vi "LJUD U3RAW Reset.vi"(7 "Comm Settings":T1={"Open LabJack "=TRUE, "Address"="1", "FirstFound"=TRUE}, 8 "error in (no error)":errorcluster, 11 "Handle In":i32) -> (0 "error out":errorcluster, 3 "Handle Out":i32)   [LabVIEW 2021]
panel:
  in  "Hard Reset":bool=TRUE
  in  "Soft Reset":bool
  out "Read Array":u8[](array[numeric]) format="%.0x"
  # "If open is false,\nthen a valid\nhandle must be\npassed in."
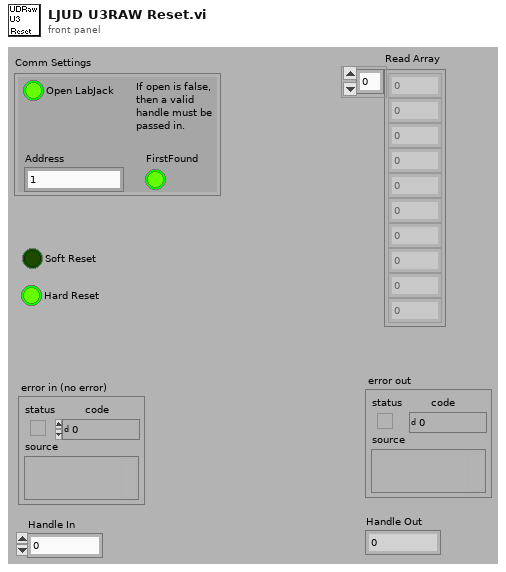
[diagram p1: front panel]
types:
  T1 = cluster{"Open LabJack ":bool, "Address":string, "FirstFound":bool}
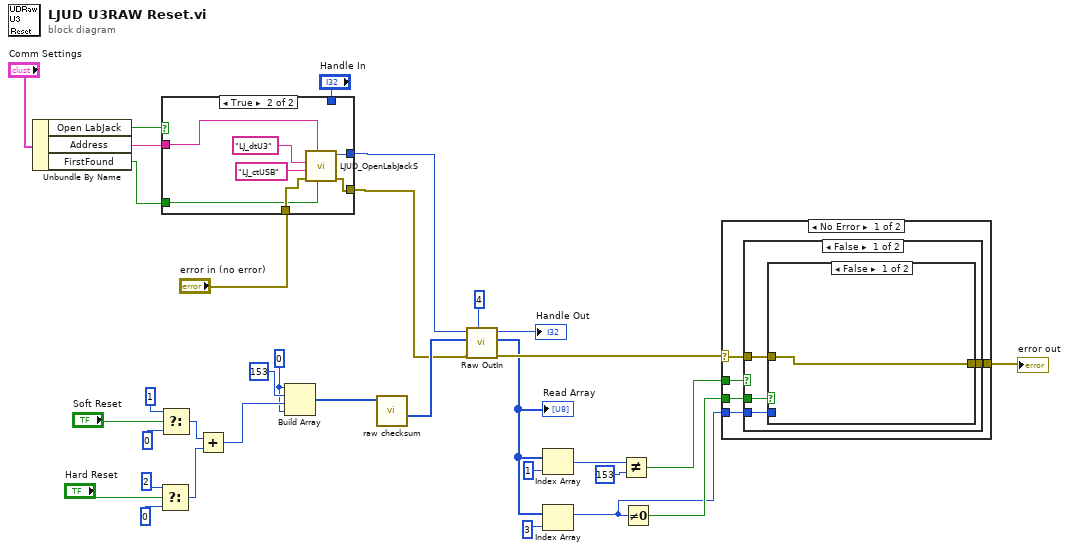
[diagram p0: block diagram]
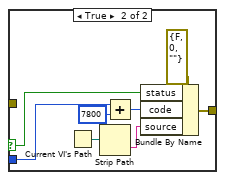
[diagram p2: hidden frame]
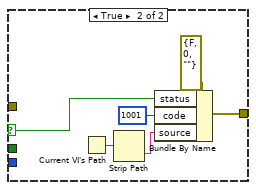
[diagram p3: hidden frame]
diagram:
  w9 = u8 0 ("Input Element")
  n1 = Unbundle By Name("Comm Settings") -> ("Open LabJack"=w23:bool, "Address"=w22:string, "FirstFound"=w21:bool)
  n2 = Select(t=u8 2 ("f"), s="Hard Reset", f=u8 0) -> (s? t:f=w12:u8)
  n3 = Select(t=u8 1 ("f"), s="Soft Reset", f=u8 0) -> (s? t:f=w11:u8)
  n4 = case shown="True" w23 {
    tunnel: w22 -> [_ w39]
    tunnel: "error in (no error)" -> [w35 w40]
    tunnel: [w35 w41] -> w26
    tunnel: [w34 w42] -> w25
    tunnel: w21 -> [_ w38]
    tunnel: "Handle In" -> [w34 _]
    frame False {
    }
    frame True {
      n5 = call "LJUD_OpenLabJackS.vi"("FirstFound"=w38, "Address"=w39, "error in"=w40, "ConnectionType"="LJ_ctUSB", "DeviceType"="LJ_dtU3") -> ("error out"=w41:errorcluster, "Handle"=w42:i32)  [unwired: 4 in, 1 out]
    }
  }
  n6 = Add(x=w11, y=w12) -> (x+y=w10:u8)
  n7 = Build Array(w9, u8 153 ("Input Element"), w10, w9) -> (w32:u8[])
  n8 = call "raw checksum.vi"("Array"=w32) -> ("Array Output"=w30:u8[])  [unwired: 3 in, 7 out]
  n9 = call "Raw OutIn.vi"("# of bytes to read in"=4 ("# of bytes to read"), "error in"=w26, "Raw Out"=w30, "Handle In"=w25) -> ("error out"=w17:errorcluster, "Raw In"=w3:u8[], "Handle Out"=→"Handle Out":i32)  [unwired: 4 in, 1 out]
  "Read Array" <- w3
  n10 = Index Array(array=w3, index=1 ("Index")) -> (element=w19:u8)
  n11 = Index Array(array=w3, index=3 ("Index")) -> (element=w1:u8)
  n12 = Not Equal?(x=w19, y=u8 153 ("Input Element")) -> (x != y?=w8:bool)
  n13 = Not Equal To 0?(x=w1) -> (x != 0?=w16:bool)
  n14 = case shown="No Error" w17 {
    selector: w17 -> [w43 w67]
    tunnel: w8 -> [w47 _]
    tunnel: w16 -> [w46 _]
    tunnel: w1 -> [w45 _]
    tunnel: [w44 w67] -> w15
    frame No Error {
      n15 = case shown="False" w47 {
        selector: w47 -> [_ w61]
        tunnel: w46 -> [w51 _]
        tunnel: w45 -> [w50 _]
        tunnel: [w49 w63] -> w44
        tunnel: w43 -> [w48 _]
        frame False {
          n16 = case shown="False" w51 {
            selector: w51 -> [_ w54]
            tunnel: w50 -> [_ w55]
            tunnel: [w52 w53] -> w49
            tunnel: w48 -> [w52 _]
            frame False {
            }
            frame True {
              n17 = Current VI's Path() -> (path=w58:path)
              n18 = Strip Path(path=w58) -> (name=w57:string)  [unwired: 1 out]
              n19 = Add(x=w55, y=7800) -> (x+y=w59:i32)
              n20 = Bundle By Name(cluster=errorcluster {"status"=FALSE, "code"=0, "source"=""} ("error IO"), "status"=w54, "code"=w59, "source"=w57) -> (w53:errorcluster)
            }
          }
        }
        frame True {
          n21 = Current VI's Path() -> (path=w66:path)
          n22 = Strip Path(path=w66) -> (name=w65:string)  [unwired: 1 out]
          n23 = Bundle By Name(cluster=errorcluster {"status"=FALSE, "code"=0, "source"=""} ("error IO"), "status"=w61, "code"=1001, "source"=w65) -> (w63:errorcluster)
        }
      }
    }
    frame Error {
    }
  }
  "error out" <- w15
